vi "parseCRC.vi"(8 "error in (no error)":errorcluster, 11 "FrameParser in":refnum<class "FrameParser.lvclass">) -> (0 "error out":errorcluster, 2 "CRC":u16, 3 "FrameParser out":refnum<class "FrameParser.lvclass">)   [LabVIEW 2015, in "FrameParser.lvclass"]
uses:
  FrameParser.lvclass
  FrameParser.lvclass/FrameParser.ctl
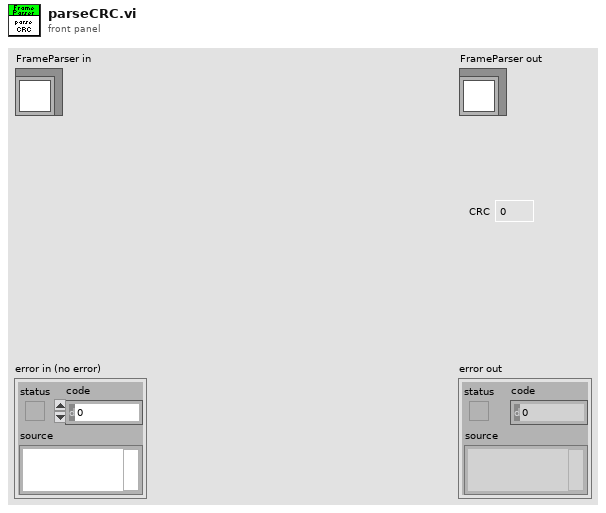
[diagram p1: front panel]
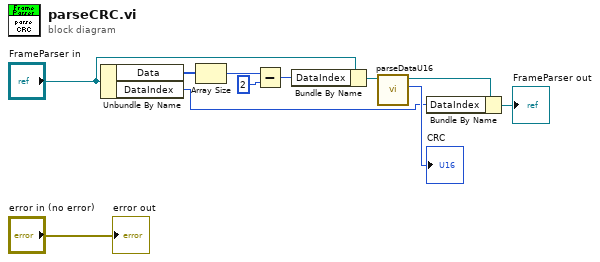
[diagram p0: block diagram]
diagram:
  n1 = Unbundle By Name("FrameParser in") -> ("Data"=w11:u8[], "DataIndex"=w3:i32)
  n2 = Array Size(array=w11) -> (size(s)=w10:i32)
  n3 = Subtract(x=w10, y=2) -> (x-y=w7:i32)
  n4 = Bundle By Name(cluster="FrameParser in", "DataIndex"=w7) -> (w6:refnum<class "FrameParser.lvclass">)
  n5 = call "parseDataU16.vi"("FrameParser in"=w6) -> ("Data"=→"CRC":u16, "FrameParser out"=w4:refnum<class "FrameParser.lvclass">)  [unwired: 8 in, 1 out]
  n6 = Bundle By Name(cluster=w4, "DataIndex"=w3) -> (→"FrameParser out":refnum<class "FrameParser.lvclass">)
  "error out" <- "error in (no error)"
